vi "ClimbRetract.vi"(11 "Button":bool) -> (3 "Complete?":bool)   [LabVIEW 2015]
panel:
  in  "Motor Power":dbl
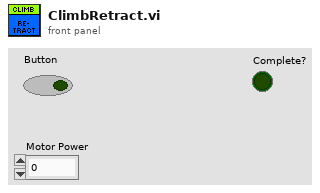
[diagram p1: front panel]
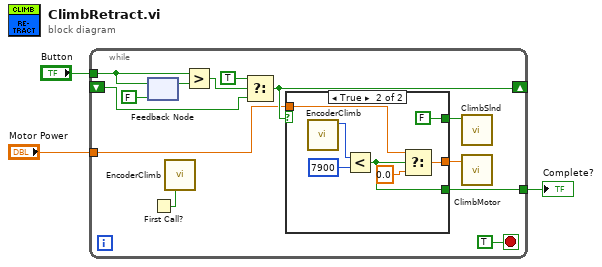
[diagram p0: block diagram]
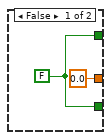
[diagram p2: hidden frame]
diagram:
  n1 = while {
    tunnel: "Button" -> [w15]
    shift-right: [w13] -> _
    shift-left: _ -> [w14]
    tunnel: [w6] -> w2
    tunnel: "Motor Power" -> [w4]
    stop <- TRUE stop-if-true
    n2 = feedback #1(FALSE) -> (w10:bool)
    n3 = feedback-in #1(w15) -> ()
    n4 = First Call?() -> (First Call?: T/F=w5:bool)
    n5 = call "EncoderClimb.vi"("Zero"=w5) -> ()  [unwired: 10 in, 1 out]
    n6 = Greater?(x=w15, y=w10) -> (0:w9:bool)
    n7 = Select(t=TRUE, s=w9, f=w14) -> (s? t:f=w13:bool)
    n8 = case shown="True" w13 {
      tunnel: [w17 FALSE] -> w12
      tunnel: [0.0 w21] -> w7
      tunnel: [w17 w20] -> w6
      tunnel: w4 -> [_ w19]
      frame False {
        w17 = FALSE
      }
      frame True {
        n9 = call "EncoderClimb.vi"() -> ("Position_out"=w25:i32)  [unwired: 11 in]
        n10 = Less?(x=w25, y=7900) -> (x < y?=w20:bool)
        n11 = Select(t=w19, s=w20, f=0.0) -> (s? t:f=w21:dbl)
      }
    }
    n12 = call "ClimbSlnd.vi"("Button"=w12) -> ()  [unwired: 11 in]
    n13 = call "ClimbMotor.vi"("Power"=w7) -> ()  [unwired: 11 in]
  }
  "Complete?" <- w2
